vi "SV Vector Average Spectra (Complex).vi"(0 "complex spectra":T7(array[cluster]) {"spectrum info"."x-axis units" items=["Time (s)"=0, "Frequency-CB (Hz)"=1, "Frequency-CPB (Hz)"=1248, "Frequency-Arbitrary (Hz)"=2357, "Quefrency (s)"=2, "Revolutions (rev)"=3, "Order"=4, "Speed (RPM)"=11, "Speed (rad/s)"=21, "Index"=65535]; "spectrum info"."weighting filter" items=["Linear", "A-weighting", "B-weighting", "C-weighting", "ITU-R 468-4", "Dolby", "CCITT", "C-message", "Wb", "Wc", "Wd", "We", "Wf", "Wh", "Wj", "Wk", "Wm", "AES17 20 kHz lowpass", "AES17 40 kHz lowpass", "AES17 20 kHz highpass", "AES17 40 kHz highpass"]; "spectrum info"."dB reference [EU]" format="%.2f"; "spectrum info"."engineering units" items=["custom..."=0, "V"=1, "A"=21, "C"=30, "pC"=31, "s"=32, "-"=29, "Pa"=2, "N"=20, "g"=3, "m/s^2"=4, "m/s"=5, "m"=6, "mm/s"=12, "mm"=13, "micron/s"=14, "micron"=15, "in/s^2"=7, "in/s"=8, "in"=9, "mil/s"=10, "mil"=11, "rad/s^2"=16, "rad/s"=17, "rad"=18, "deg/s^2"=26, "deg/s"=27, "deg"=28, "RPM"=22, "cycle/s^2"=23, "Hz"=24, "cycle"=25, "strain"=19]; "spectrum info"."spectral info"."window" items=["None "=0, "Hanning"=1, "Hamming"=2, "Blackman-Harris"=3, "Exact Blackman"=4, "Blackman"=5, "Flat Top"=6, "4 Term B-Harris "=7, "7 Term B-Harris"=8, "Low Sidelobe"=9, "Force - Exponential"=10, "Gaussian"=62]; "complex spectrum response"."complex spectrum" format="%.2f"; "complex spectrum response"."df" format="%.2f"; "complex spectrum response"."f0" format="%.2f"}, 5 "error in (no error)":errorcluster) -> (13 "averages completed":dbl, 14 "vector average complex spectrum":T8={"complex spectrum response"={"f0"=0.0, "df"=1.0, "complex spectrum"=[]}, "spectrum info"={"channel name"="", "description"="", "x-axis units"=0, "spectral info"={"spectrum type"=enum."Power [Magnitude^2]", "linear/dB"=enum."linear", "window"=0, "window size"=0, "FFT size"=0}, "engineering units"=0, "custom label"="", "dB reference [EU]"=0.0, "peak units"=enum."rms", "weighting filter"=0, "spectral density?"=FALSE, "unit label"="", "spectrum skewed?"=FALSE, "complimentary spectrum units"=enum."none"}} {"spectrum info"."x-axis units" items=["Time (s)"=0, "Frequency-CB (Hz)"=1, "Frequency-CPB (Hz)"=1248, "Frequency-Arbitrary (Hz)"=2357, "Quefrency (s)"=2, "Revolutions (rev)"=3, "Order"=4, "Speed (RPM)"=11, "Speed (rad/s)"=21, "Index"=65535]; "spectrum info"."weighting filter" items=["Linear", "A-weighting", "B-weighting", "C-weighting", "ITU-R 468-4", "Dolby", "CCITT", "C-message", "Wb", "Wc", "Wd", "We", "Wf", "Wh", "Wj", "Wk", "Wm", "AES17 20 kHz lowpass", "AES17 40 kHz lowpass", "AES17 20 kHz highpass", "AES17 40 kHz highpass"]; "spectrum info"."dB reference [EU]" format="%.2f"; "spectrum info"."engineering units" items=["custom..."=0, "V"=1, "A"=21, "C"=30, "pC"=31, "s"=32, "-"=29, "Pa"=2, "N"=20, "g"=3, "m/s^2"=4, "m/s"=5, "m"=6, "mm/s"=12, "mm"=13, "micron/s"=14, "micron"=15, "in/s^2"=7, "in/s"=8, "in"=9, "mil/s"=10, "mil"=11, "rad/s^2"=16, "rad/s"=17, "rad"=18, "deg/s^2"=26, "deg/s"=27, "deg"=28, "RPM"=22, "cycle/s^2"=23, "Hz"=24, "cycle"=25, "strain"=19]; "spectrum info"."spectral info"."window" items=["None "=0, "Hanning"=1, "Hamming"=2, "Blackman-Harris"=3, "Exact Blackman"=4, "Blackman"=5, "Flat Top"=6, "4 Term B-Harris "=7, "7 Term B-Harris"=8, "Low Sidelobe"=9, "Force - Exponential"=10, "Gaussian"=62]; "complex spectrum response"."complex spectrum" format="%.2f"; "complex spectrum response"."df" format="%.2f"; "complex spectrum response"."f0" format="%.2f"}, 19 "error out":errorcluster)   [LabVIEW 2017]
doc: "Computes the linear vector-averaged spectrum of <b>complex spectra</b>. Use vector averaging to reduce uncorrelated component levels in the average spectra in order to quantify correlated signal components as a function of frequency."
uses:
  <vilib>/addons/_NISVFA/_Shared subVIs/Controls/svc_Spectrum Info.ctl
  <vilib>/addons/_NISVFA/_Shared subVIs/Controls/svc_X-Axis Units.ctl
  <vilib>/addons/_NISVFA/_Shared subVIs/Controls/svc_Spectrum Type.ctl
  <vilib>/addons/_NISVFA/_Shared subVIs/Controls/svc_Engineering Units Text Ring.ctl
  <vilib>/addons/_NISVFA/_Shared subVIs/Controls/svc_Weighting Filter Text Ring.ctl
  <vilib>/addons/_NISVFA/_Shared subVIs/Controls/svc_Complimentary Spectrum Units.ctl
  <vilib>/addons/_NISVFA/_Shared subVIs/Common/sv_Get NI Property Name String.vi
  <vilib>/addons/_NISVFA/_Shared subVIs/Spectrum Info/sfva_Set SV Info in Spectrum Info Description.vi
  <vilib>/addons/_NISVFA/_Shared subVIs/Spectrum Info/sfva_Get SV Info from Spectrum Info Description.vi
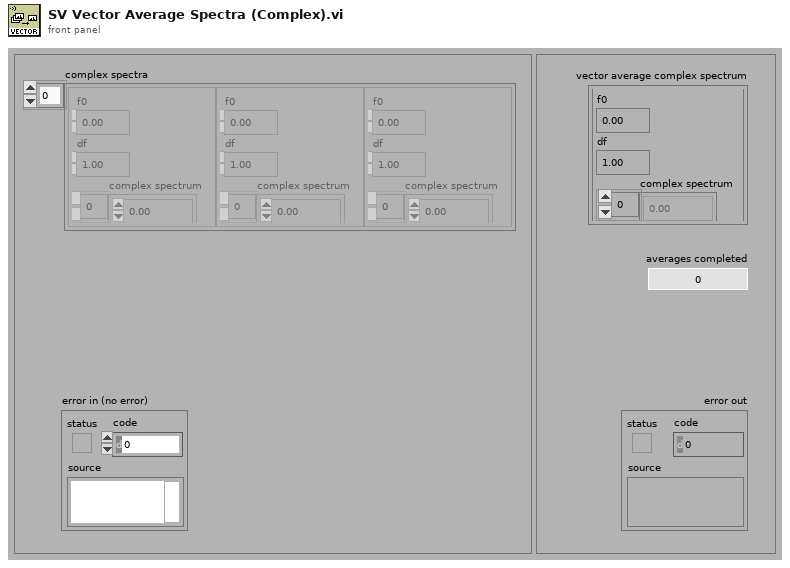
[diagram p1: front panel]
types:
  T1 = typedef "svc_Spectrum Info.ctl" = cluster{"channel name":string, "description":string, "x-axis units":T2, "spectral info":cluster{"spectrum type":T3, "linear/dB":enum16{"linear", "dB"}, "window":u16, "window size":i32, "FFT size":i32}, "engineering units":T4, "custom label":string, "dB reference [EU]":dbl, "peak units":enum16{"rms", "peak", "peak-peak"}, "weighting filter":T5, "spectral density?":bool, "unit label":string, "spectrum skewed?":bool, "complimentary spectrum units":T6}
  T2 = typedef "svc_X-Axis Units.ctl" = u16
  T3 = typedef "svc_Spectrum Type.ctl" = enum16{"FFT Spectrum [complex]", "Amplitude [Magnitude]", "Power [Magnitude^2]", "Cross Spectrum [complex]", "Frequency Response [Complex]"}
  T4 = typedef "svc_Engineering Units Text Ring.ctl" = u16
  T5 = typedef "svc_Weighting Filter Text Ring.ctl" = u16
  T6 = typedef "svc_Complimentary Spectrum Units.ctl" = enum16{"none", "radians", "degrees", "cycles", "imaginary"}
  T7 = cluster{"complex spectrum response":cluster{"f0":dbl, "df":dbl, "complex spectrum":cdb[]}, "spectrum info":T1}[]
  T8 = cluster{"complex spectrum response":cluster{"f0":dbl, "df":dbl, "complex spectrum":cdb[]}, "spectrum info":T1}
  T9 = enum16{"No averaging", "Vector averaging", "RMS averaging", "Peak hold"}
  T10 = enum16{"No averaging", "Vector averaging", "RMS averaging", "Peak hold"}[]
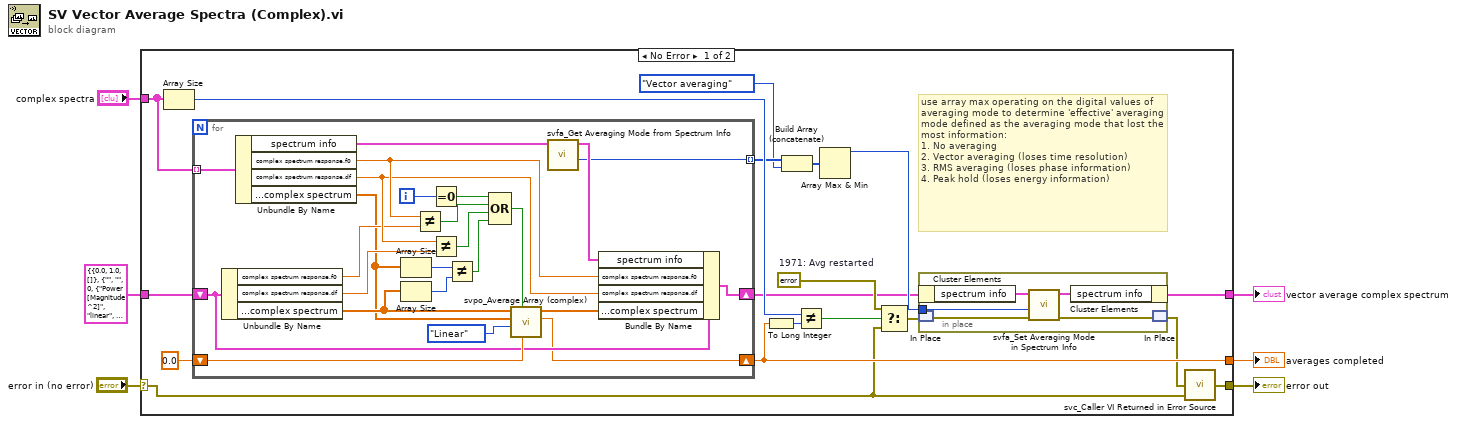
[diagram p0: block diagram]
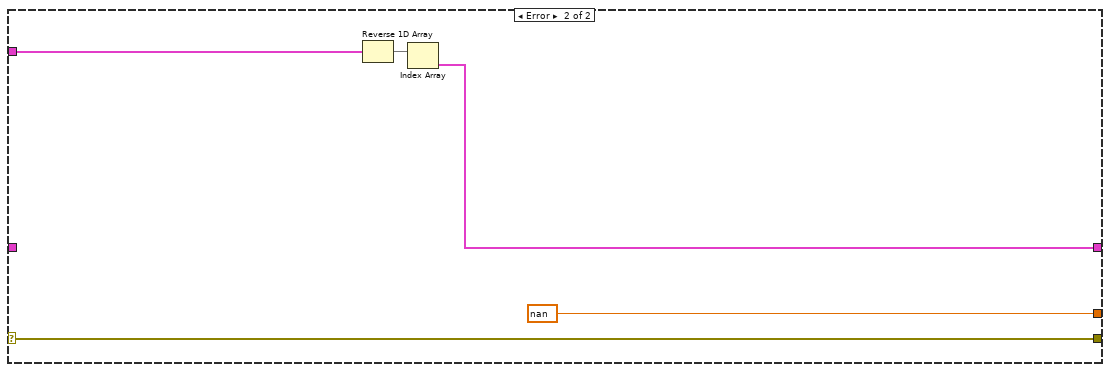
[diagram p2: hidden frame]
diagram:
  n1 = case shown="No Error" "error in (no error)" {
    selector: "error in (no error)" -> [w15 w57]
    tunnel: [w8 w54] -> w1
    tunnel: "complex spectra" -> [w17 w56]
    tunnel: [w23 nan ("Numeric")] -> w4
    tunnel: [w18 w57] -> w3
    tunnel: T8 {"complex spectrum response"={"f0"=0.0, "df"=1.0, "complex spectrum"=[]}, "spectrum info"={"channel name"="", "description"="", "x-axis units"=0, "spectral info"={"spectrum type"=enum."Power [Magnitude^2]", "linear/dB"=enum."linear", "window"=0, "window size"=0, "FFT size"=0}, "engineering units"=0, "custom label"="", "dB reference [EU]"=0.0, "peak units"=enum."rms", "weighting filter"=0, "spectral density?"=FALSE, "unit label"="", "spectrum skewed?"=FALSE, "complimentary spectrum units"=enum."none"}} ("complex spectrum") -> [w16 _]
    frame No Error {
      w20 = errorcluster {"status"=FALSE, "code"=1971, "source"="<append>\nAveraging restarted due to change in f0, df, or spectrum size within complex spectra input."}  # 1971: Avg restarted
      # "use array max operating on the digital values of averaging mode to determine 'effective' averaging mode defined as the averaging mode that lost the most information:\n1. No averaging \n2. Vector averaging (loses time resolution)\n3. RMS averaging (loses phase information)\n4. Peak hold (loses energy information)"
      n2 = Array Size(array=w17) -> (size(s)=w22:i32)
      n3 = for {
        tunnel: w17 -> [w36] mode=indexing
        shift-right: [w39] -> w23
        shift-left: 0.0 ("Numeric") -> [w47]
        shift-right: [w40] -> w10
        shift-left: w16 -> [w44]
        tunnel: [w32] -> w13 mode=indexing
        i -> [w45]
        n4 = Unbundle By Name(w44) -> ("complex spectrum response.f0"=w38:dbl, "complex spectrum response.df"=w37:dbl, "complex spectrum response.complex spectrum"=w31:cdb[])
        n5 = Unbundle By Name(w36) -> ("spectrum info"=w35:T1, "complex spectrum response.f0"=w42:dbl, "complex spectrum response.df"=w41:dbl, "complex spectrum response.complex spectrum"=w30:cdb[])
        n6 = Array Size(array=w30) -> (size(s)=w53:i32)
        n7 = Array Size(array=w31) -> (size(s)=w52:i32)
        n8 = Not Equal?(x=w42, y=w38) -> (x != y?=w51:bool)
        n9 = Equal To 0?(x=w45) -> (x = 0?=w46:bool)
        n10 = Not Equal?(x=w41, y=w37) -> (x != y?=w49:bool)
        n11 = Not Equal?(x=w53, y=w52) -> (x != y?=w50:bool)
        n12 = Compound Arithmetic op=OR(w46, w51, w49, w50) -> (w34:bool)
        n13 = call <vilib>:"svpo_Average Array (complex).vi"("averages completed in"=w47, "restart averaging"=w34, "weighting mode"=enum16{"Linear", "Exponential"}."Linear", "array"=w30, "previous average array"=w31) -> ("averages completed out"=w39:dbl, "average array"=w43:cdb[])  [unwired: 5 in]
        n14 = call <vilib>:"svfa_Get Averaging Mode from Spectrum Info.vi"("spectrum info"=w35) -> ("averaging mode"=w32:T9, "spectrum info"=w33:T1)  [unwired: 8 in, 1 out]
        n15 = Bundle By Name(cluster=w44, "spectrum info"=w33, "complex spectrum response.f0"=w42, "complex spectrum response.df"=w41, "complex spectrum response.complex spectrum"=w43) -> (w40:T8)
      }
      n16 = To Long Integer(number=w23) -> (32bit integer=w21:i32)
      n17 = Build Array (concatenate)(w13, T9."Vector averaging" ("averaging mode")) -> (w14:T10)
      n18 = Not Equal?(x=w22, y=w21) -> (x != y?=w19:bool)
      n19 = Array Max & Min(array=w14) -> (max value=w11:T9)  [unwired: 3 out]
      n20 = Select(t=w20, s=w19, f=w15) -> (s? t:f=w9:errorcluster)
      n21 = in-place {
        in-place-border: w11 -> [w29]
        n22 = in-place-cluster #1(w10) -> ("spectrum info"=w28:T1)
        n23 = in-place-match #2(w9) -> (w27:errorcluster)
        n24 = call <vilib>:"svfa_Set Averaging Mode in Spectrum Info.vi"("error in"=w27, "averaging mode"=w29, "spectrum info in"=w28) -> ("error out"=w26:errorcluster, "spectrum info out"=w25:T1)  [unwired: 7 in]
        n25 = in-place-cluster #1("spectrum info"=w25) -> (w8:T8)
        n26 = in-place-match #2(w26) -> (w7:errorcluster)
      }
      n27 = call <vilib>:"svc_Caller VI Returned in Error Source.vi"("warning input to caller"=w15, "error in (no error)"=w7) -> ("error out"=w18:errorcluster)  [unwired: 3 in]
    }
    frame Error {
      n28 = Reverse 1D Array(array=w56) -> (reversed array=w55:T7)
      n29 = Index Array(array=w55) -> (element=w54:T8)  [unwired: 1 in]
    }
  }
  "vector average complex spectrum" <- w1
  "averages completed" <- w4
  "error out" <- w3
